vi "Programa 01.vi"() -> ()   [LabVIEW 2013]
uses:
  <vilib>/Instr/_visa.llb/VISA Configure Serial Port (Instr).vi
panel:
  out "Estado":dbl
  in  "Velocidad M2":bool
  in  "FPGA Leds":bool
  in  "Giro M2":bool
  in  "FPGA Leds 2":bool
  out "= Run":bool
  in  "Always: Stop":bool
  in  "Always: Start":bool
  out "Contrarrelog":bool
  out "Relog":bool
  out "11":bool
  out "12":bool
  out "13":bool
  out "14":bool
  in  "stop":bool
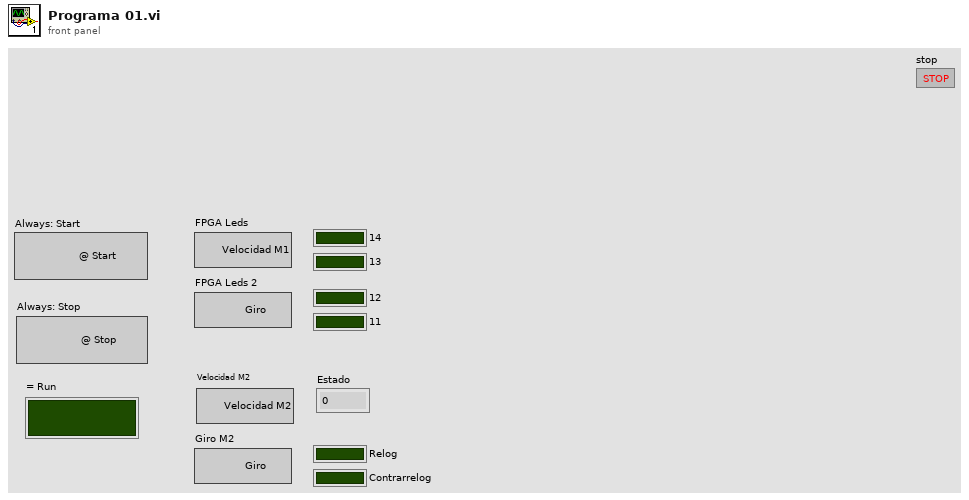
[diagram p1: front panel]
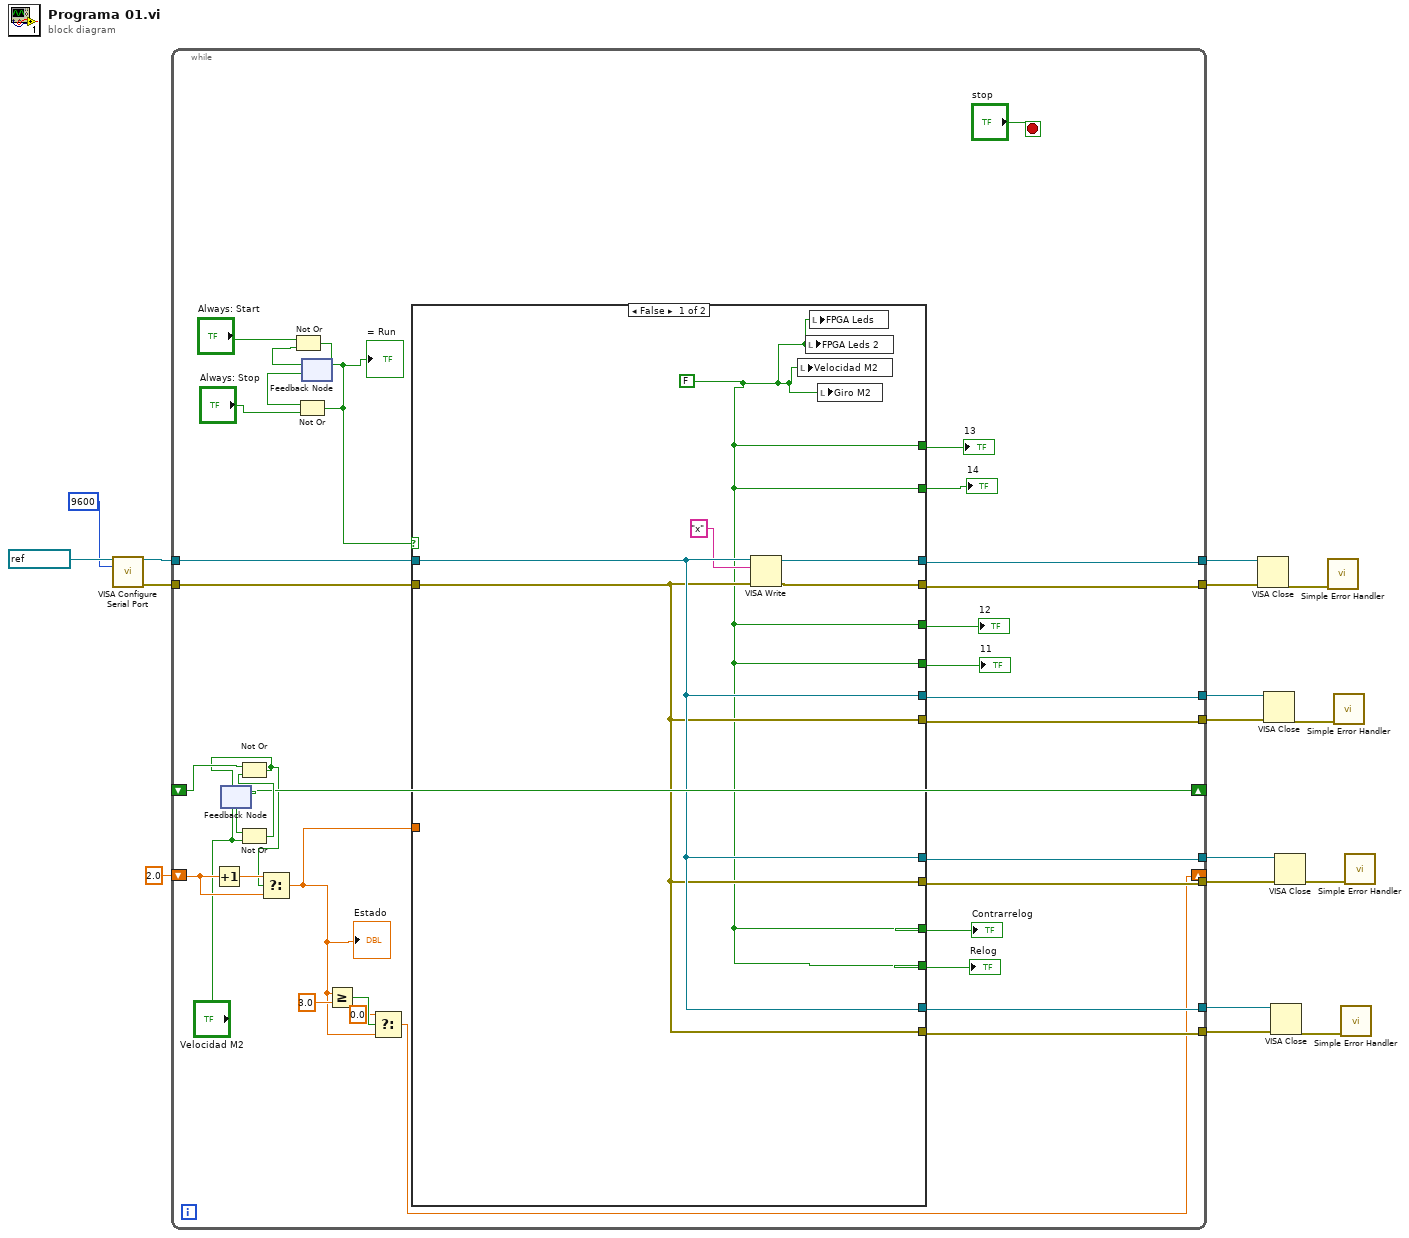
[diagram p0: block diagram]
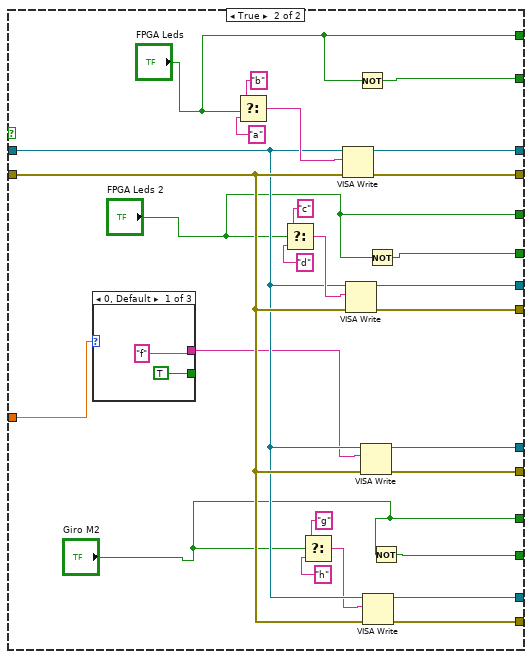
[diagram p2: hidden frame]
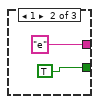
[diagram p3: hidden frame]
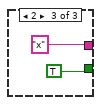
[diagram p4: hidden frame]
diagram:
  n1 = call-poly "VISA Configure Serial Port"("VISA resource name"=refnum<visa-resource-name> "COM6", "baud rate (9600)"=u32 9600) -> ("VISA resource name out"=w14:refnum<visa-resource-name>, "error out"=w13:errorcluster)  [unwired: 12 in]
  n2 = while {
    tunnel: [w48] -> w16
    tunnel: [w47] -> w15
    tunnel: w14 -> [w46]
    tunnel: w13 -> [w45]
    tunnel: [w42] -> w11
    tunnel: [w41] -> w10
    tunnel: [w38] -> w7
    tunnel: [w37] -> w6
    tunnel: [w36] -> w5
    tunnel: [w35] -> w4
    shift-right: ["Velocidad M2"] -> _
    shift-left: _ -> [w25]
    shift-right: [w22] -> _
    shift-left: 2.0 -> [w28]
    stop <- "stop" stop-if-true
    n3 = Increment(x=w28) -> (x+1=w29:dbl)
    n4 = feedback #1() -> (w26:bool)  [unwired: 1 in]
    n5 = Not Or(1:"Velocidad M2", 2:w26) -> (0:w27:bool)
    n6 = Not Or(1:w27, 2:w25) -> (0:w18:bool)
    n7 = feedback-in #1(w18) -> ()
    n8 = Select(t=w29, s=w18, f=w28) -> (s? t:f=w19:dbl)
    "Estado" <- w19
    n9 = feedback #2() -> (w49:bool)  [unwired: 1 in]
    n10 = Not Or(1:w49, 2:"Always: Start") -> (0:w50:bool)
    n11 = Not Or(1:"Always: Stop", 2:w50) -> (0:w30:bool)
    "= Run" <- w30
    n12 = feedback-in #2(w30) -> ()
    n13 = Greater Or Equal?(x=w19, y=3.0) -> (x >= y?=w24:bool)
    n14 = Select(t=0.0, s=w24, f=w19) -> (s? t:f=w22:dbl)
    n15 = case shown="False" w30 {
      tunnel: [w57 w84] -> w48
      tunnel: [w56 w83] -> w47
      tunnel: w46 -> [w55 w71]
      tunnel: w45 -> [w54 w72]
      tunnel: [w52 w79] -> w44
      tunnel: [w52 "FPGA Leds"] -> w43
      tunnel: [w55 w78] -> w42
      tunnel: [w54 w77] -> w41
      tunnel: [w52 w73] -> w40
      tunnel: [w52 "FPGA Leds 2"] -> w39
      tunnel: [w55 w70] -> w38
      tunnel: [w54 w69] -> w37
      tunnel: [w55 w68] -> w36
      tunnel: [w54 w67] -> w35
      tunnel: [w52 w66] -> w34
      tunnel: [w52 "Giro M2"] -> w33
      tunnel: w19 -> [_ w59]
      frame False {
        w52 = FALSE
        n16 = VISA Write(VISA resource name=w55, write buffer="x", error in (no error)=w54) -> (VISA resource name out=w57:refnum<visa-resource-name>, error out=w56:errorcluster)  [unwired: 1 out]
        n17 = local write "Velocidad M2"(w52) -> ()
        n18 = local write "FPGA Leds 2"(w52) -> ()
        n19 = local write "FPGA Leds"(w52) -> ()
        n20 = local write "Giro M2"(w52) -> ()
      }
      frame True {
        n21 = case shown="0, Default" w59 {
          tunnel: ["f" "e" "x"] -> w58
          tunnel: [TRUE TRUE TRUE] -> _
          frame 0, Default {
          }
          frame 1 {
          }
          frame 2 {
          }
        }
        n22 = Select(t="b", s="FPGA Leds", f="a") -> (s? t:f=w80:string)
        n23 = Select(t="c", s="FPGA Leds 2", f="d") -> (s? t:f=w74:string)
        n24 = Select(t="g", s="Giro M2", f="h") -> (s? t:f=w63:string)
        n25 = VISA Write(VISA resource name=w71, write buffer=w80, error in (no error)=w72) -> (VISA resource name out=w84:refnum<visa-resource-name>, error out=w83:errorcluster)  [unwired: 1 out]
        n26 = VISA Write(VISA resource name=w71, write buffer=w74, error in (no error)=w72) -> (VISA resource name out=w78:refnum<visa-resource-name>, error out=w77:errorcluster)  [unwired: 1 out]
        n27 = Not(x="FPGA Leds") -> (.not. x?=w79:bool)
        n28 = VISA Write(VISA resource name=w71, write buffer=w58, error in (no error)=w72) -> (VISA resource name out=w70:refnum<visa-resource-name>, error out=w69:errorcluster)  [unwired: 1 out]
        n29 = VISA Write(VISA resource name=w71, write buffer=w63, error in (no error)=w72) -> (VISA resource name out=w68:refnum<visa-resource-name>, error out=w67:errorcluster)  [unwired: 1 out]
        n30 = Not(x="FPGA Leds 2") -> (.not. x?=w73:bool)
        n31 = Not(x="Giro M2") -> (.not. x?=w66:bool)
      }
    }
    "13" <- w43
    "14" <- w44
    "12" <- w39
    "11" <- w40
    "Relog" <- w34
    "Contrarrelog" <- w33
  }
  n32 = VISA Close(VISA resource name=w16, error in (no error)=w15) -> (error out=w17:errorcluster)
  n33 = VISA Close(VISA resource name=w11, error in (no error)=w10) -> (error out=w12:errorcluster)
  n34 = VISA Close(VISA resource name=w5, error in (no error)=w4) -> (error out=w8:errorcluster)
  n35 = VISA Close(VISA resource name=w7, error in (no error)=w6) -> (error out=w9:errorcluster)
  n36 = call <vilib>:"Simple Error Handler.vi"("error in (no error)"=w17) -> ()  [unwired: 4 in, 5 out]
  n37 = call <vilib>:"Simple Error Handler.vi"("error in (no error)"=w12) -> ()  [unwired: 4 in, 5 out]
  n38 = call <vilib>:"Simple Error Handler.vi"("error in (no error)"=w8) -> ()  [unwired: 4 in, 5 out]
  n39 = call <vilib>:"Simple Error Handler.vi"("error in (no error)"=w9) -> ()  [unwired: 4 in, 5 out]
